vi "ByViServerInterfaceTemplate_4x4x4_CreateClass.vi"(1 "ProjectTreePosition(String or Project Item Ref)":variant, 2 "CreateClassData":T1, 3 "ClassTemplateFolder":path, 5 "error in (no error)":errorcluster, 6 "KeepLvClassRefOpen(False)":bool, 7 "HeaderToApply (take from VIRef or /use 2D-8bit header, Ignored if not wired)":variant) -> (15 "LVClassLibraryRefnum":refnum<vi>, 16 "TemplateVersionUsed":string, 19 "error out":errorcluster)   [LabVIEW 2012]
uses:
  <resource>/Framework/Providers/Open_GDS/ClassProviders/Provider_BaseClassInterface/CreateClassData.ctl
  <resource>/Framework/Providers/Open_GDS/ClassProviders/Common/LvClass_class/GDSLvCLass_ClassSettingsType.ctl
  <resource>/Framework/Providers/Open_GDS/ClassProviders/Common/LvClass_class/GDSLvClass_PlugIn.ctl
  <resource>/Framework/Providers/Open_GDS/ClassProviders/Common/LvClass_class/GDSLvClass_PlugInTypes.ctl
  <resource>/Framework/Providers/Open_GDS/ClassProviders/Provider_BaseClassInterface/ClassWriter_class/ClassWriter.lvclass
  <resource>/Framework/Providers/Open_GDS/ClassProviders/Provider_EndevoGOOP400/ClassWriterGOOP400_class/ClassWriterGOOP400.lvclass
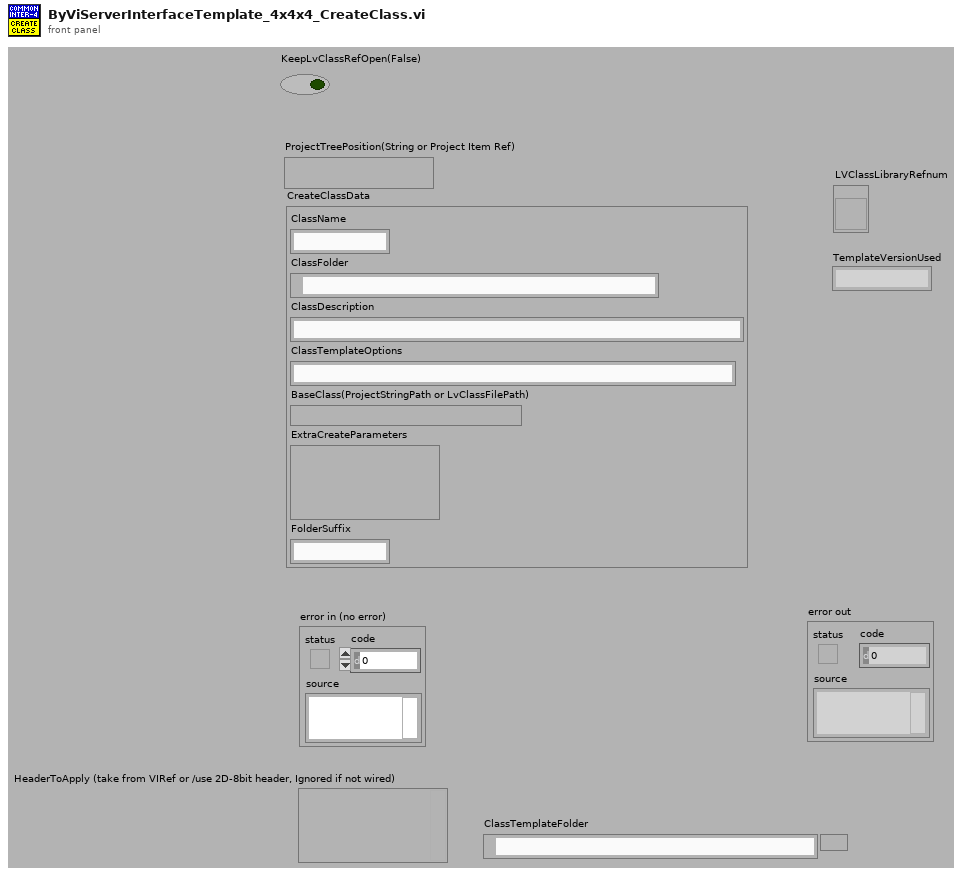
[diagram p1: front panel]
types:
  T1 = typedef "ClassWriter.lvclass/CreateClassData.ctl" = cluster{"ClassName":string, "ClassFolder":path, "ClassDescription":string, "ClassTemplateOptions":string, "BaseClass(ProjectStringPath or LvClassFilePath)":variant, "ExtraCreateParameters":variant, "FolderSuffix":string}
  T2 = cluster{"SubClass":bool, "ClassTemplateFiles":path[], "ClassName":string, "ClassFolder":path, "VIs":refnum<vi>[], "TemplateFolder":path, "ViSubDirs":string[], "TemplateName":string, "BaseClassFolder":path, "RootBaseClassFolder":path, "LvClassPath":path, "ClassRefnum":refnum<vi>, "ProjectRefnum":refnum<vi>, "LvClassFolderPath":path, "BaseClassName":string, "ClassItems":refnum<vi>[], "ViLocked":bool[], "ProjectItemOwner":refnum<vi>, "DeleteFiles":path[], "VIsBefore":refnum<vi>[], "BaseClassPath":path, "BaseConstructorBase":path, "TemplBaseConstructorBase":path, "TemplatePath":path, "TemplateVersion":string, "TemplateParentClass":refnum<vi>, "App":refnum<vi>, "Parent Class":refnum<vi>, "ParentVIs":refnum<vi>[], "TempClass":refnum<vi>}
  T3 = typedef "GDSLvCLass_ClassSettingsType.ctl" = cluster{"ClassProviderName":string, "ClassTemplateUsed":string, "ClassTemplateVersion":string, "ClassDescription":string, "PlugIns":T4[], "ConnectorPanePattern":string}
  T4 = typedef "GDSLvClass_PlugIn.ctl" = cluster{"Type":T5, "ID":string, "Version":string, "Path":path, "Name":string, "Data":variant}
  T5 = typedef "GDSLvClass_PlugInTypes.ctl" = enum16{"DesignPattern", "MethodTypes"}
  T6 = enum32{"invalid lock state", "Not Locked", "Locked (No Password)", "Password-protected"}
  T7 = cluster{"Major":u16, "Minor":u16, "Fix":u16, "Build":u16}
  T8 = typedef "Scripting_ConnectorPanePatternType.ctl" = u16
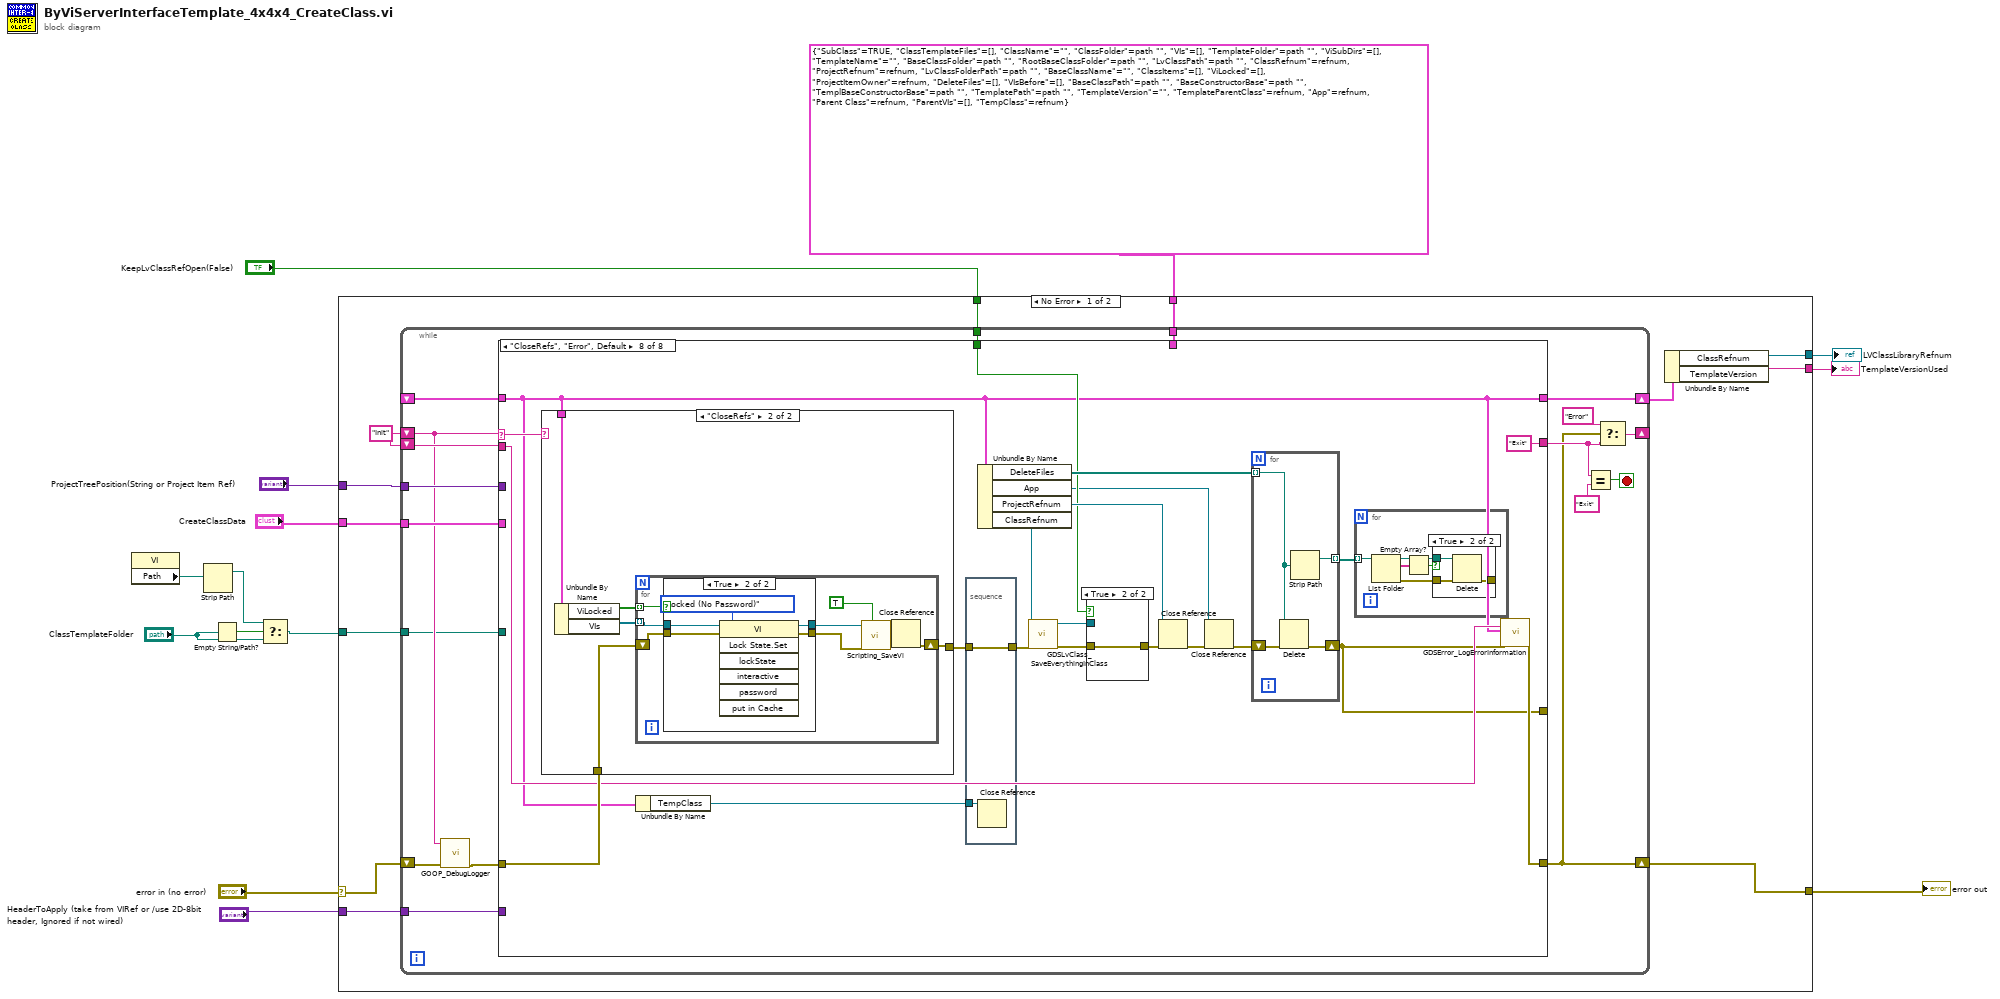
[diagram p0: block diagram]
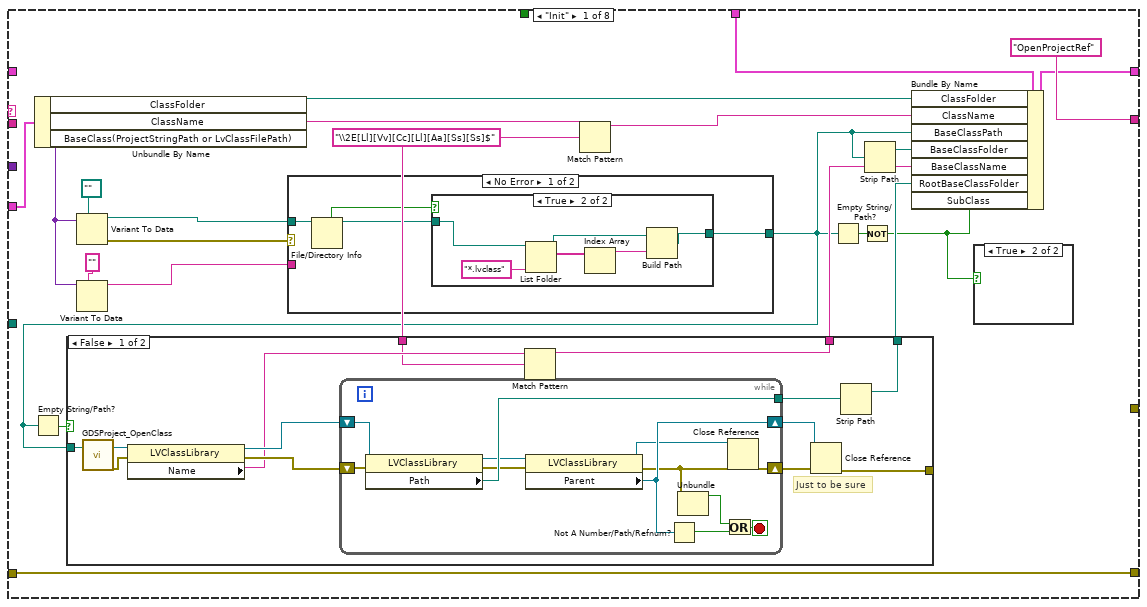
[diagram p2: hidden frame]
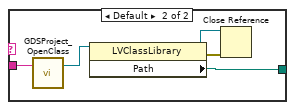
[diagram p7: hidden frame]
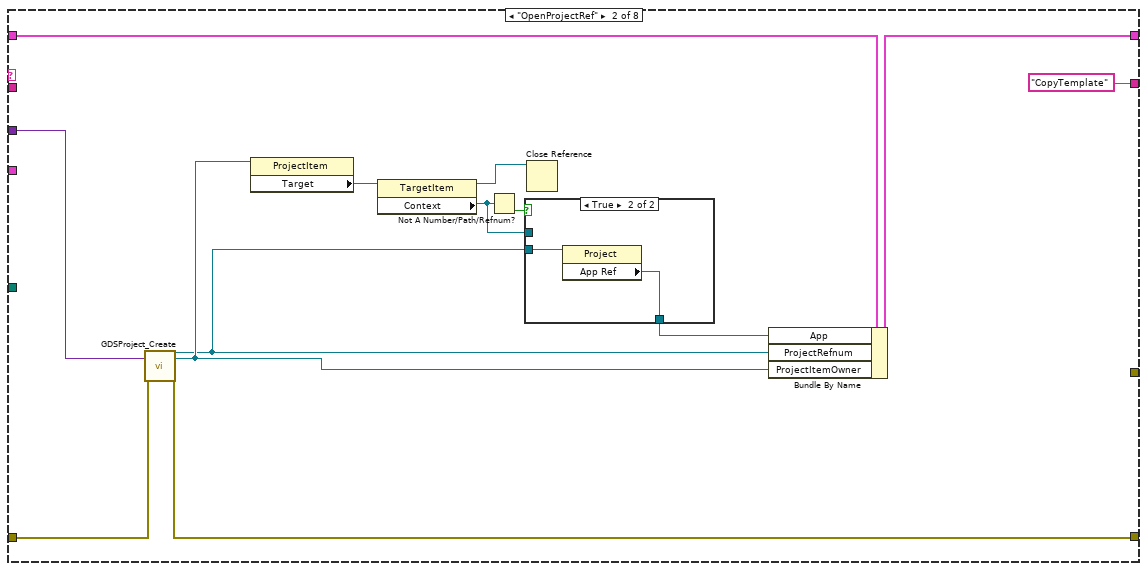
[diagram p8: hidden frame]
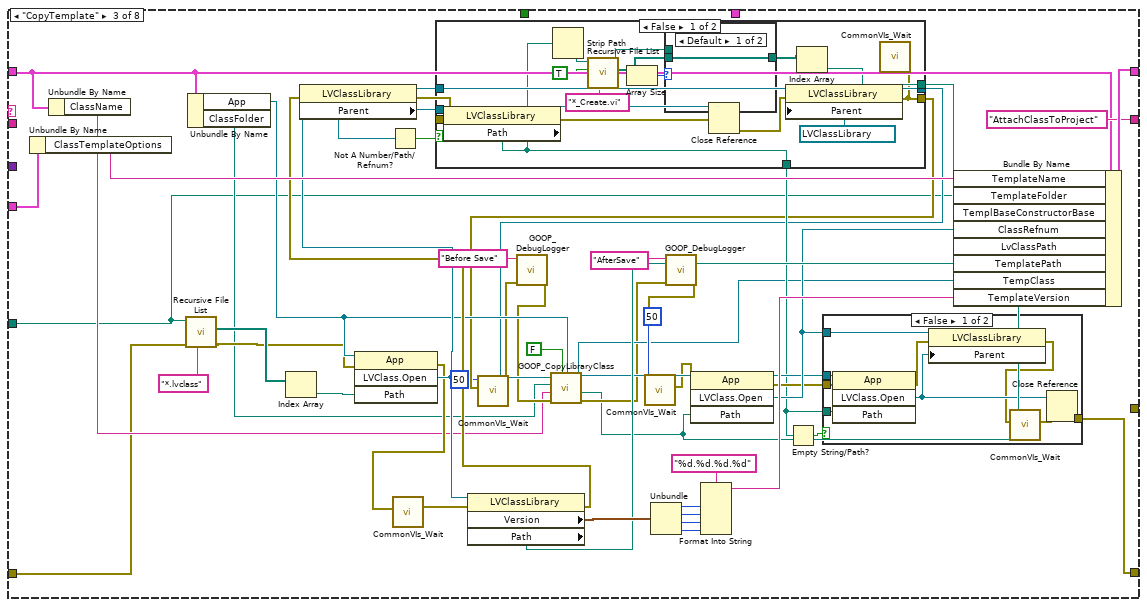
[diagram p10: hidden frame]
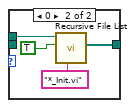
[diagram p12: hidden frame]
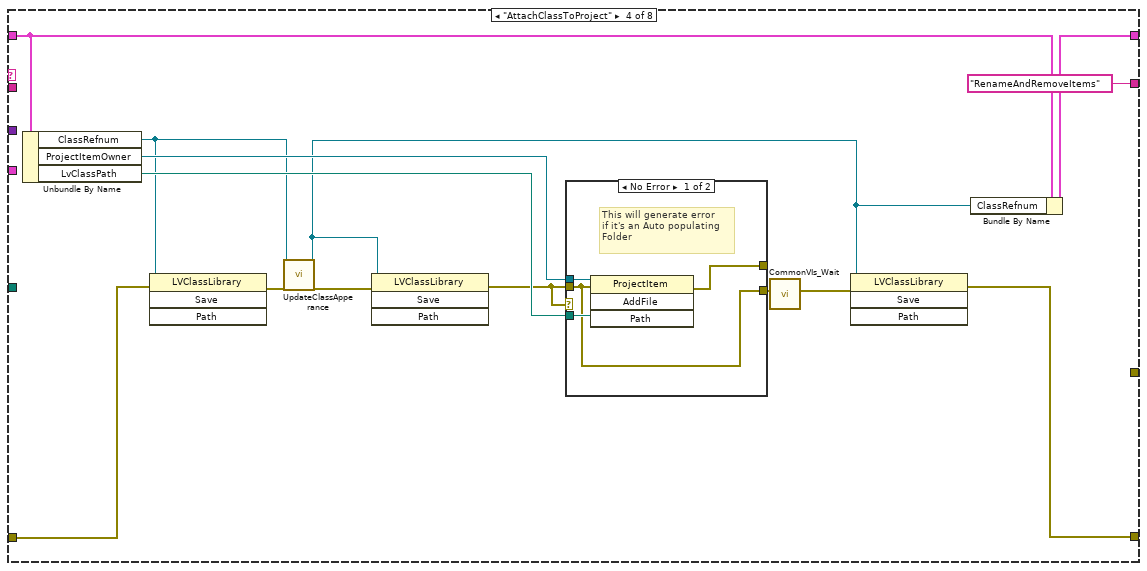
[diagram p14: hidden frame]
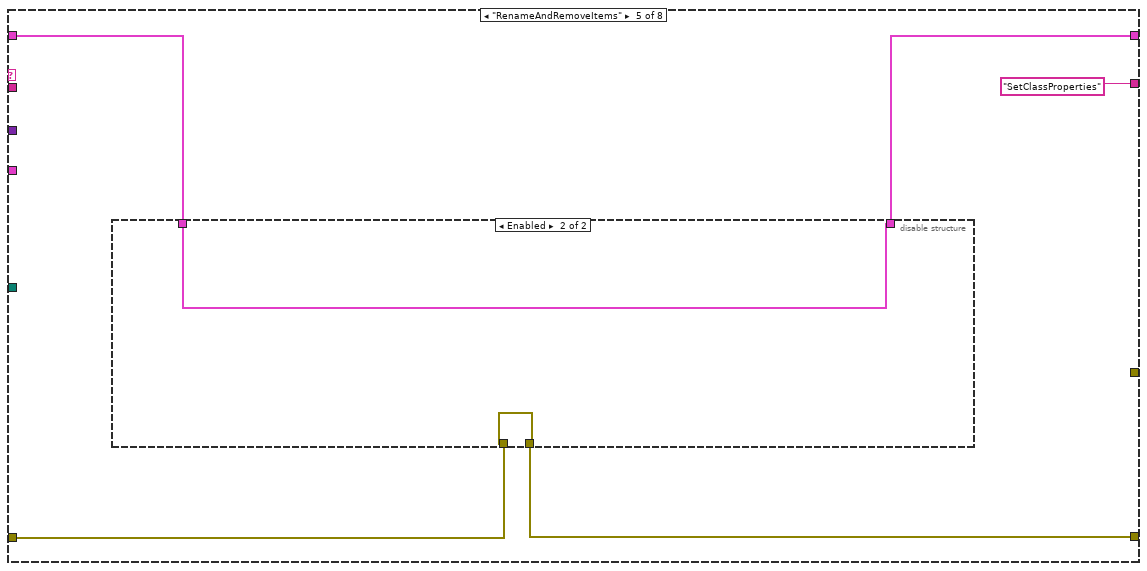
[diagram p16: hidden frame]
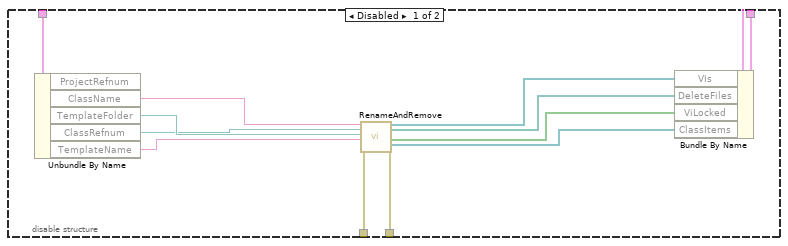
[diagram p17: hidden frame]
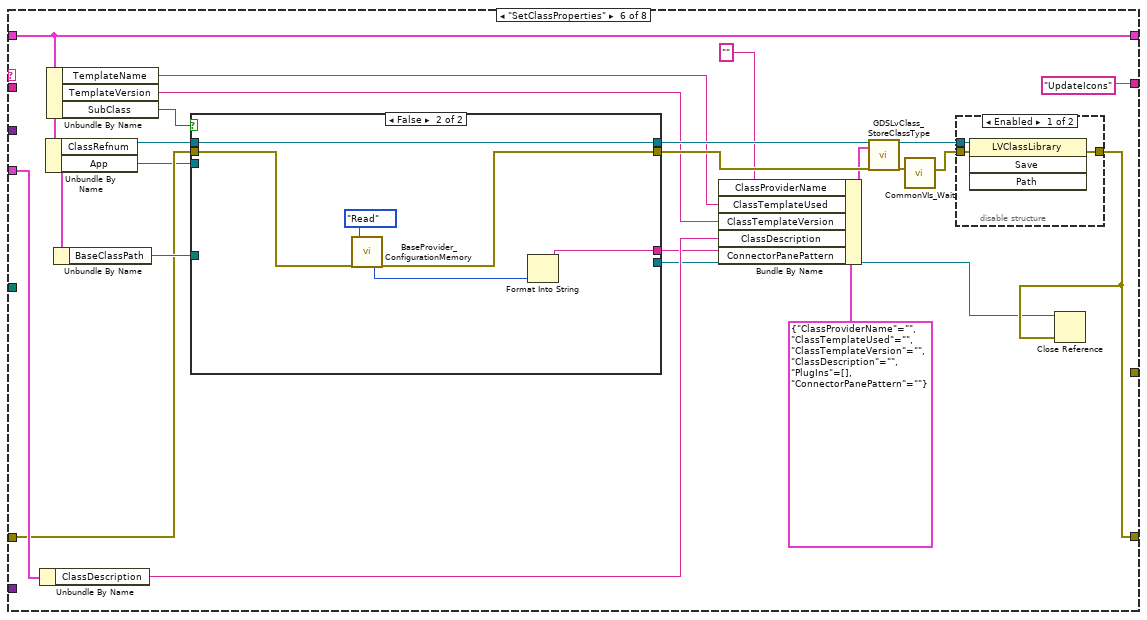
[diagram p18: hidden frame]
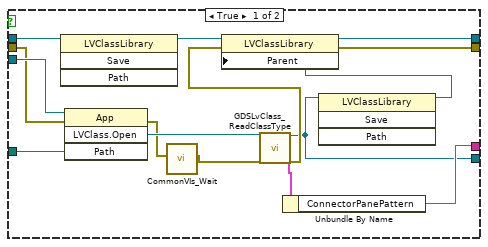
[diagram p20: hidden frame]
diagram:
  n1 = property class="VI"() -> ("Path"=w5:path)  [unwired: 2 in, 2 out]
  n2 = Strip Path(path=w5) -> (stripped path=w2:path)  [unwired: 1 out]
  n3 = Empty String/Path?(string/path="ClassTemplateFolder") -> (empty?=w4:bool)
  n4 = Select(t=w2, s=w4, f="ClassTemplateFolder") -> (s? t:f=w1:path)
  n5 = case shown="No Error" "error in (no error)" {
    selector: "error in (no error)" -> [w17 w368]
    tunnel: [w26 w368] -> w12
    tunnel: "ProjectTreePosition(String or Project Item Ref)" -> [w25 _]
    tunnel: "CreateClassData" -> [w24 _]
    tunnel: "HeaderToApply (take from VIRef or /use 2D-8bit header, Ignored if not wired)" -> [w23 _]
    tunnel: "KeepLvClassRefOpen(False)" -> [w22 _]
    tunnel: [w21 _] -> w7
    tunnel: [w20 _] -> w6
    tunnel: T2 {"SubClass"=TRUE, "ClassTemplateFiles"=[], "ClassName"="", "ClassFolder"=path "", "VIs"=[], "TemplateFolder"=path "", "ViSubDirs"=[], "TemplateName"="", "BaseClassFolder"=path "", "RootBaseClassFolder"=path "", "LvClassPath"=path "", "ClassRefnum"=refnum, "ProjectRefnum"=refnum, "LvClassFolderPath"=path "", "BaseClassName"="", "ClassItems"=[], "ViLocked"=[], "ProjectItemOwner"=refnum, "DeleteFiles"=[], "VIsBefore"=[], "BaseClassPath"=path "", "BaseConstructorBase"=path "", "TemplBaseConstructorBase"=path "", "TemplatePath"=path "", "TemplateVersion"="", "TemplateParentClass"=refnum, "App"=refnum, "Parent Class"=refnum, "ParentVIs"=[], "TempClass"=refnum} ("output cluster") -> [w19 _]
    tunnel: w1 -> [w15 _]
    frame No Error {
      w16 = "Init" ("t")
      n6 = while {
        shift-right: [w36] -> w26
        shift-left: w17 -> [w30]
        shift-right: [w40] -> _
        shift-left: w16 -> [w28]
        shift-right: [w43] -> w18
        shift-left: _ -> [w44]
        tunnel: w19 -> [w38]
        tunnel: w25 -> [w35]
        tunnel: w24 -> [w34]
        shift-left: w16 -> [w33]
        tunnel: w23 -> [w32]
        tunnel: w22 -> [w31]
        tunnel: w15 -> [w27]
        stop <- w41 stop-if-true
        n7 = call <resource>:"GOOP_DebugLogger.vi"("error in (no error)"=w30, "State"=w28) -> ("error out"=w29:errorcluster)  [unwired: 9 in]
        n8 = case shown="\"CloseRefs\", \"Error\", Default" w28 {
          selector: w28 -> [_ _ _ _ _ _ _ w323]
          tunnel: w44 -> [_ w120 w170 w223 w233 w259 w303 w307]
          tunnel: [w63 w119 w175 w222 w234 w259 w303 w307] -> w43
          tunnel: w29 -> [w66 w118 w125 w217 w231 w260 w297 w324]
          tunnel: [w66 w116 w145 w213 w232 w251 w298 w320] -> w36
          tunnel: ["OpenProjectRef" "CopyTemplate" "AttachClassToProject" "RenameAndRemoveItems" "SetClassProperties" "UpdateIcons" "CloseRefs" "Exit"] -> w37
          tunnel: w38 -> [w59 _ _ _ _ _ _ _]
          tunnel: w35 -> [_ w117 _ _ _ _ _ _]
          tunnel: w34 -> [w58 _ w169 _ _ w266 _ _]
          tunnel: w33 -> [_ _ _ _ _ _ _ w319]
          tunnel: w32 -> [_ _ _ _ _ _ w301 _]
          tunnel: w31 -> [_ _ _ _ _ _ _ w315]
          tunnel: [_ _ _ _ _ _ _ w313] -> _
          tunnel: w27 -> [_ _ w126 _ _ _ _ _]
          frame "Init" {
            w55 = "\\2E[Ll][Vv][Cc][Ll][Aa][Ss][Ss]$" ("regular expression")
            n9 = Unbundle By Name(w58) -> ("ClassFolder"=w52:path, "ClassName"=w51:string, "BaseClass(ProjectStringPath or LvClassFilePath)"=w57:variant)
            n10 = Variant To Data(type=path "" ("path"), Variant=w57) -> (data=w48:path, error out=w49:errorcluster)  [unwired: 1 in]
            n11 = Variant To Data(type="" ("regular expression"), Variant=w57) -> (data=w60:string)  [unwired: 1 in, 1 out]
            n12 = case shown="No Error" w49 {
              tunnel: [w94 w102] -> w46
              tunnel: w60 -> [_ w103]
              tunnel: w48 -> [w93 _]
              frame No Error {
                n13 = File/Directory Info(path=w93) -> (path out=w91:path, directory=w92:bool)  [unwired: 1 in, 5 out]
                n14 = case shown="True" w92 {
                  tunnel: [w95 w97] -> w94
                  tunnel: w91 -> [w95 w96]
                  frame False {
                  }
                  frame True {
                    n15 = List Folder(path=w96, pattern="*.lvclass") -> (path out=w98:path, filenames=w100:string[])  [unwired: 2 in, 2 out]
                    n16 = Index Array(array=w100) -> (element=w99:string)  [unwired: 1 in]
                    n17 = Build Path(base path=w98, name or relative path=w99) -> (appended path=w97:path)
                  }
                }
              }
              frame Error {
                n18 = case shown="\"\"" w103 {
                  tunnel: w103 -> [_ w108]
                  tunnel: [_ w104] -> w102
                  frame "" {
                  }
                  frame Default {
                    n19 = call <resource>:"GDSProject_OpenClass.vi"("ClassPath(FilePath/ProjectTreePath/LvCLassRef)"=w108) -> ("LVClass.Open"=w107:refnum<vi>)  [unwired: 16 in, 2 out]
                    n20 = property class="LVClassLibrary"(reference=w107) -> (reference out=w105:refnum<vi>, error out=w106:errorcluster, "Path"=w104:path)  [unwired: 1 in]
                    n21 = Close Reference(reference=w105, error in (no error)=w106) -> ()  [unwired: 1 out]
                  }
                }
              }
            }
            n22 = Empty String/Path?(string/path=w46) -> (empty?=w53:bool)
            n23 = case shown="False" w53 {
              tunnel: [w76 _] -> w56
              tunnel: w55 -> [w70 _]
              tunnel: [w69 _] -> w54
              tunnel: w46 -> [w68 _]
              tunnel: [w67 _] -> _
              frame False {
                # "Just to be sure"
                n24 = call <resource>:"GDSProject_OpenClass.vi"("ClassPath(FilePath/ProjectTreePath/LvCLassRef)"=w68) -> ("LVClass.Open"=w73:refnum<vi>, "error out"=w75:errorcluster)  [unwired: 16 in, 1 out]
                n25 = property class="LVClassLibrary"(reference=w73, error in=w75) -> (reference out=w72:refnum<vi>, error out=w74:errorcluster, "Name"=w71:string)
                n26 = while {
                  shift-right: [w87] -> w79
                  shift-left: w74 -> [w82]
                  shift-right: [w88] -> w78
                  shift-left: w72 -> [w90]
                  tunnel: [w89] -> w77
                  stop <- w84 stop-if-true
                  n27 = property class="LVClassLibrary"(reference=w90, error in=w82) -> (reference out=w80:refnum<vi>, error out=w81:errorcluster, "Path"=w89:path)
                  n28 = property class="LVClassLibrary"(reference=w80, error in=w81) -> (reference out=w83:refnum<vi>, error out=w87:errorcluster, "Parent"=w88:refnum<vi>)
                  n29 = Not A Number/Path/Refnum?(number/path/refnum=w88) -> (NaN/Path/Refnum?=w85:bool)
                  n30 = Unbundle(w87) -> ("status"=w86:bool)  [unwired: 2 out]
                  n31 = Or(x=w86, y=w85) -> (x .or. y?=w84:bool)
                  n32 = Close Reference(reference=w83) -> ()  [unwired: 1 in, 1 out]
                }
                n33 = Match Pattern(string=w71, regular expression=w70) -> (before substring=w69:string)  [unwired: 1 in, 3 out]
                n34 = Close Reference(reference=w78, error in (no error)=w79) -> (error out=w67:errorcluster)
                n35 = Strip Path(path=w77) -> (stripped path=w76:path)  [unwired: 1 out]
              }
              frame True {
              }
            }
            n36 = Match Pattern(string=w51, regular expression=w55) -> (before substring=w64:string)  [unwired: 1 in, 3 out]
            n37 = Empty String/Path?(string/path=w46) -> (empty?=w47:bool)
            n38 = Not(x=w47) -> (.not. x?=w45:bool)
            n39 = Strip Path(path=w46) -> (stripped path=w50:path)  [unwired: 1 out]
            n40 = Bundle By Name(cluster=w59, "ClassFolder"=w52, "ClassName"=w64, "BaseClassPath"=w46, "BaseClassFolder"=w50, "BaseClassName"=w54, "RootBaseClassFolder"=w56, "SubClass"=w45) -> (w63:T2)
            n41 = case shown="True" w45 {
              frame False {
              }
              frame True {
              }
            }
          }
          frame "OpenProjectRef" {
            n42 = call <resource>:"GDSProject_Create.vi"("ProjectTreePosition(String or Project Item Ref)"=w117, "error in (no error)"=w118) -> ("Project Refnum"=w110:refnum<vi>, "Project Item"=w111:refnum<vi>, "error out"=w116:errorcluster)  [unwired: 15 in]
            n43 = property class="ProjectItem"(reference=w111) -> ("Target"=w115:refnum<vi>)  [unwired: 1 in, 2 out]
            n44 = property class="TargetItem"(reference=w115) -> (reference out=w114:refnum<vi>, "Context"=w112:refnum<vi>)  [unwired: 1 in, 1 out]
            n45 = Not A Number/Path/Refnum?(number/path/refnum=w112) -> (NaN/Path/Refnum?=w113:bool)
            n46 = case shown="True" w113 {
              tunnel: [w122 w124] -> w109
              tunnel: w110 -> [_ w123]
              tunnel: w112 -> [w122 _]
              frame False {
              }
              frame True {
                n47 = property class="Project"(reference=w123) -> ("App Ref"=w124:refnum<vi>)  [unwired: 1 in, 2 out]
              }
            }
            n48 = Close Reference(reference=w114) -> ()  [unwired: 1 in, 1 out]
            n49 = Bundle By Name(cluster=w120, "App"=w109, "ProjectRefnum"=w110, "ProjectItemOwner"=w111) -> (w119:T2)
          }
          frame "CopyTemplate" {
            n50 = Unbundle By Name(w169) -> ("ClassTemplateOptions"=w168:string)
            n51 = Unbundle By Name(w170) -> ("ClassName"=w129:string)
            n52 = call <vilib>:"Recursive File List.vi"("pattern"="*.lvclass", "error in (no error)"=w125, "Folder Path"=w126) -> ("error out"=w146:errorcluster, "All Files in Dir"=w172:path[])  [unwired: 4 in, 3 out]
            n53 = Unbundle By Name(w170) -> ("App"=w147:refnum<vi>, "ClassFolder"=w128:path)
            n54 = Index Array(array=w172) -> (element=w171:path)  [unwired: 1 in]
            n55 = invoke class="App" method="LVClass.Open"(reference=w147, error in=w146, "Path"=w171) -> (error out=w142:errorcluster, "LVClass.Open"=w154:refnum<vi>)  [unwired: 1 in, 2 out]
            n56 = call <resource>:"CommonVIs_Wait.vi"("error in"=w142) -> ("error out"=w143:errorcluster)  [unwired: 9 in]
            n57 = property class="LVClassLibrary"(reference=w154, error in=w143) -> (error out=w155:errorcluster, "Version"=w167:T7, "Path"=w161:path)  [unwired: 1 out]
            n58 = property class="LVClassLibrary"(reference=w154, error in=w155) -> (reference out=w159:refnum<vi>, error out=w151:errorcluster, "Parent"=w152:refnum<vi>)
            n59 = Not A Number/Path/Refnum?(number/path/refnum=w152) -> (NaN/Path/Refnum?=w150:bool)
            n60 = case shown="False" w150 {
              tunnel: w159 -> [w200 w209]
              tunnel: [w199 w209] -> w133
              tunnel: [w186 w210] -> w141
              tunnel: [w196 _] -> w153
              tunnel: w152 -> [w194 _]
              tunnel: w151 -> [w193 w210]
              tunnel: [w191 _] -> w149
              frame False {
                n61 = property class="LVClassLibrary"(reference=w194, error in=w193) -> (reference out=w202:refnum<vi>, error out=w203:errorcluster, "Path"=w191:path)
                n62 = Strip Path(path=w191) -> (stripped path=w195:path)  [unwired: 1 out]
                n63 = call <vilib>:"Recursive File List.vi"("pattern"="*_Create.vi", "Treat LLBs as Folders?"=TRUE, "Folder Path"=w195) -> ("All Files in Dir"=w187:path[], "dup Folder Path"=w188:path)  [unwired: 4 in, 3 out]
                n64 = Array Size(array=w187) -> (size(s)=w190:i32)
                n65 = case shown="Default" w190 {
                  tunnel: w187 -> [w204 _]
                  tunnel: [w204 w205] -> w189
                  tunnel: w188 -> [_ w206]
                  frame Default {
                  }
                  frame 0 {
                    n66 = call <vilib>:"Recursive File List.vi"("pattern"="*_Init.vi", "Treat LLBs as Folders?"=TRUE, "Folder Path"=w206) -> ("All Files in Dir"=w205:path[])  [unwired: 4 in, 4 out]
                  }
                }
                n67 = Close Reference(reference=w202, error in (no error)=w203) -> (error out=w201:errorcluster)
                n68 = property class="LVClassLibrary"(reference=w200, error in=w201, "Parent"=refnum<vi> refnum ("Parent Class")) -> (reference out=w199:refnum<vi>, error out=w186:errorcluster)
                n69 = Index Array(array=w189) -> (element=w196:path)  [unwired: 1 in]
                n70 = call <resource>:"CommonVIs_Wait.vi"("error in"=w186) -> ()  [unwired: 9 in, 1 out]
              }
              frame True {
              }
            }
            n71 = call <resource>:"CommonVIs_Wait.vi"("error in"=w141, "Wait(150ms)"=u32 50) -> ("error out"=w138:errorcluster)  [unwired: 8 in]
            n72 = call <resource>:"GOOP_DebugLogger.vi"("error in (no error)"=w138, "State"="Before Save") -> ("error out"=w132:errorcluster)  [unwired: 9 in]
            n73 = call <resource>:"GOOP_CopyLibraryClass.vi"("ManualCopy"=FALSE, "error in"=w132, "New Name"=w129, "Path"=w128, "LVClassIn"=w133) -> ("error out"=w131:errorcluster, "New Lib Path"=w130:path, "LVClassOut"=w134:refnum<vi>)  [unwired: 4 in]
            n74 = Unbundle(w167) -> ("Major"=w165:u16, "Minor"=w164:u16, "Fix"=w163:u16, "Build"=w162:u16)
            n75 = call <resource>:"GOOP_DebugLogger.vi"("error in (no error)"=w131, "State"="AfterSave") -> ("error out"=w136:errorcluster)  [unwired: 9 in]
            n76 = call <resource>:"CommonVIs_Wait.vi"("error in"=w136, "Wait(150ms)"=u32 50) -> ("error out"=w144:errorcluster)  [unwired: 8 in]
            n77 = invoke class="App" method="LVClass.Open"(reference=w147, error in=w144, "Path"=w130) -> (reference out=w157:refnum<vi>, error out=w156:errorcluster, "LVClass.Open"=w158:refnum<vi>)  [unwired: 1 in, 1 out]
            n78 = Format Into String(format string="%d.%d.%d.%d", w165, w164, w163, w162) -> (resulting string=w160:string)  [unwired: 2 in, 1 out]
            n79 = Empty String/Path?(string/path=w149) -> (empty?=w148:bool)
            n80 = case shown="False" w148 {
              tunnel: w158 -> [w184 _]
              tunnel: w157 -> [w183 _]
              tunnel: w156 -> [w182 w185]
              tunnel: [w181 w185] -> w145
              tunnel: w149 -> [w179 _]
              frame False {
                n81 = invoke class="App" method="LVClass.Open"(reference=w183, error in=w182, "Path"=w179) -> (error out=w178:errorcluster, "LVClass.Open"=w180:refnum<vi>)  [unwired: 1 in, 2 out]
                n82 = property class="LVClassLibrary"(reference=w184, error in=w178, "Parent"=w180) -> (error out=w176:errorcluster)  [unwired: 1 out]
                n83 = call <resource>:"CommonVIs_Wait.vi"("error in"=w176) -> ("error out"=w177:errorcluster)  [unwired: 9 in]
                n84 = Close Reference(reference=w180, error in (no error)=w177) -> (error out=w181:errorcluster)
              }
              frame True {
              }
            }
            n85 = Bundle By Name(cluster=w170, "TemplateName"=w168, "TemplateFolder"=w126, "TemplBaseConstructorBase"=w153, "ClassRefnum"=w158, "LvClassPath"=w130, "TemplatePath"=w161, "TempClass"=w134, "TemplateVersion"=w160) -> (w175:T2)
          }
          frame "AttachClassToProject" {
            n86 = Unbundle By Name(w223) -> ("ClassRefnum"=w216:refnum<vi>, "ProjectItemOwner"=w224:refnum<vi>, "LvClassPath"=w220:path)
            n87 = invoke class="LVClassLibrary" method="Save"(reference=w216, error in=w217) -> (error out=w218:errorcluster)  [unwired: 2 in, 3 out]
            n88 = call <resource>:"UpdateClassApperance.vi"("ClassRefIn"=w216, "error in (no error)"=w218) -> ("ClassRefOut"=w211:refnum<vi>, "error out"=w215:errorcluster)  [unwired: 16 in]
            n89 = invoke class="LVClassLibrary" method="Save"(reference=w211, error in=w215) -> (error out=w212:errorcluster)  [unwired: 2 in, 3 out]
            n90 = case shown="No Error" w212 {
              tunnel: w224 -> [w228 _]
              tunnel: w220 -> [w227 _]
              tunnel: [w226 w229] -> w219
              tunnel: w212 -> [w226 w229]
              tunnel: [w225 _] -> _
              frame No Error {
                # "This will generate error\nif it's an Auto populating\nFolder"
                n91 = invoke class="ProjectItem" method="AddFile"(reference=w228, error in=w226, "Path"=w227) -> (error out=w225:errorcluster)  [unwired: 1 in, 3 out]
              }
              frame Error {
              }
            }
            n92 = call <resource>:"CommonVIs_Wait.vi"("error in"=w219) -> ("error out"=w214:errorcluster)  [unwired: 9 in]
            n93 = invoke class="LVClassLibrary" method="Save"(reference=w211, error in=w214) -> (error out=w213:errorcluster)  [unwired: 2 in, 3 out]
            n94 = Bundle By Name(cluster=w223, "ClassRefnum"=w211) -> (w222:T2)
          }
          frame "RenameAndRemoveItems" {
            n95 = disable-structure shown="Enabled" {
              disable-tunnel: [w244 w247] -> w234
              disable-tunnel: w233 -> [w242 w247]
              disable-tunnel: [w240 w248] -> w232
              disable-tunnel: w231 -> [w239 w248]
              frame Disabled {
                n96 = Unbundle By Name(w242) -> ("ClassName"=w246:string, "TemplateFolder"=w243:path, "ClassRefnum"=w241:refnum<vi>, "TemplateName"=w235:string)  [unwired: 1 out]
                n97 = call <resource>:"RenameAndRemove.vi"("ClassName"=w246, "ClassRefnum"=w241, "TemplateFolder"=w243, "TemplateName"=w235, "error in"=w239) -> ("ViRefsOut"=w245:refnum<vi>[], "DeleteFiles"=w238:path[], "ItemLocked"=w237:bool[], "Items"=w236:refnum<vi>[], "error out"=w240:errorcluster)  [unwired: 10 in]
                n98 = Bundle By Name(cluster=w242, "VIs"=w245, "DeleteFiles"=w238, "ViLocked"=w237, "ClassItems"=w236) -> (w244:T2)
              }
              frame Enabled {
              }
            }
          }
          frame "SetClassProperties" {
            n99 = Unbundle By Name(w266) -> ("ClassDescription"=w263:string)
            n100 = Unbundle By Name(w259) -> ("ClassRefnum"=w261:refnum<vi>, "App"=w256:refnum<vi>)
            n101 = Unbundle By Name(w259) -> ("TemplateName"=w262:string, "TemplateVersion"=w257:string, "SubClass"=w270:bool)
            n102 = Unbundle By Name(w259) -> ("BaseClassPath"=w269:path)
            n103 = case shown="False" w270 {
              tunnel: w261 -> [w278 w295]
              tunnel: [w289 w295] -> w268
              tunnel: w260 -> [w282 w291]
              tunnel: [w288 w290] -> w267
              tunnel: w269 -> [w287 _]
              tunnel: w256 -> [w283 _]
              tunnel: [w284 w292] -> w255
              tunnel: [w276 _] -> w250
              frame True {
                n104 = invoke class="LVClassLibrary" method="Save"(reference=w278) -> (reference out=w277:refnum<vi>)  [unwired: 3 in, 3 out]
                n105 = invoke class="App" method="LVClass.Open"(reference=w283, error in=w282, "Path"=w287) -> (error out=w281:errorcluster, "LVClass.Open"=w286:refnum<vi>)  [unwired: 1 in, 2 out]
                n106 = call <resource>:"CommonVIs_Wait.vi"("error in"=w281) -> ("error out"=w280:errorcluster)  [unwired: 9 in]
                n107 = call <resource>:"GDSLvClass_ReadClassType.vi"("Class Refnum In"=w286, "error in (no error)"=w280) -> ("Class Refnum Out"=w276:refnum<vi>, "ClassSettings"=w285:T3, "error out"=w279:errorcluster)  [unwired: 15 in]
                n108 = Unbundle By Name(w285) -> ("ConnectorPanePattern"=w284:string)
                n109 = invoke class="LVClassLibrary" method="Save"(reference=w276) -> (reference out=w275:refnum<vi>)  [unwired: 3 in, 3 out]
                n110 = property class="LVClassLibrary"(reference=w277, error in=w279, "Parent"=w275) -> (reference out=w289:refnum<vi>, error out=w288:errorcluster)
              }
              frame False {
                n111 = call <resource>:"BaseProvider_ConfigurationMemory.vi"("error in (no error)"=w291, "Action"=enum16{"Read", "Load", "Save"}."Read") -> ("PatternOut"=w294:T8, "error out"=w290:errorcluster)  [unwired: 11 in, 5 out]
                n112 = Format Into String(w294) -> (resulting string=w292:string)  [unwired: 3 in, 1 out]
              }
            }
            n113 = Bundle By Name(cluster=T3 {"ClassProviderName"="", "ClassTemplateUsed"="", "ClassTemplateVersion"="", "ClassDescription"="", "PlugIns"=[], "ConnectorPanePattern"=""} ("ClassSettings"), "ClassProviderName"="", "ClassTemplateUsed"=w262, "ClassTemplateVersion"=w257, "ClassDescription"=w263, "ConnectorPanePattern"=w255) -> (w264:T3)
            n114 = call <resource>:"GDSLvClass_StoreClassType.vi"("Class Refnum In"=w268, "ClassSettings"=w264, "error in (no error)"=w267) -> ("Class Refnum Out"=w254:refnum<vi>, "error out"=w253:errorcluster)  [unwired: 15 in]
            n115 = call <resource>:"CommonVIs_Wait.vi"("error in"=w253) -> ("error out"=w252:errorcluster)  [unwired: 9 in]
            n116 = disable-structure shown="Enabled" {
              disable-tunnel: [w273 w274] -> w251
              disable-tunnel: w254 -> [w272 _]
              disable-tunnel: w252 -> [w271 w274]
              frame Enabled {
                n117 = invoke class="LVClassLibrary" method="Save"(reference=w272, error in=w271) -> (error out=w273:errorcluster)  [unwired: 2 in, 3 out]
              }
              frame Disabled {
              }
            }
            n118 = Close Reference(reference=w250, error in (no error)=w251) -> ()  [unwired: 1 out]
          }
          frame "UpdateIcons" {
            n119 = Unbundle By Name(w303) -> ("ClassRefnum"=w302:refnum<vi>)
            n120 = Unbundle By Name(w303) -> ("ClassName"=w304:string)  [unwired: 1 out]
            n121 = Empty String/Path?(string/path=w301) -> (empty?=w300:bool)
            n122 = Not(x=w300) -> (.not. x?=w299:bool)
            n123 = call <resource>:"GDSLvIcon_DialogUpdateClass.vi"("ClassPath(FilePath/ProjectTreePath/LvCLassRef)"=w302, "ClassName"=w304, "AutoUpdate"=w299, "error in (no error)"=w297, "HeaderToApply (take from VIRef or /use 2D-8bit header, Ignored if not wired)"=w301) -> ("error out"=w298:errorcluster)  [unwired: 14 in]
          }
          frame "CloseRefs", "Error", Default {
            n124 = case shown="\"CloseRefs\"" w323 {
              tunnel: w324 -> [w346 w350]
              tunnel: w307 -> [w345 w349]
              tunnel: [w346 w348] -> w308
              frame "False", Default {
                n125 = Unbundle By Name(w345) -> ("VIs"=w344:refnum<vi>[])
                n126 = Close Reference(reference=w344) -> ()  [unwired: 1 in, 1 out]
              }
              frame "CloseRefs" {
                n127 = Unbundle By Name(w349) -> ("ViLocked"=w347:bool[], "VIs"=w351:refnum<vi>[])
                n128 = for {
                  tunnel: w351 -> [w356] mode=indexing
                  shift-right: [w352] -> w348
                  shift-left: w350 -> [w357]
                  tunnel: w347 -> [w353] mode=indexing
                  n129 = case shown="True" w353 {
                    tunnel: w357 -> [w361 w367]
                    tunnel: w356 -> [w362 w366]
                    tunnel: [w361 w365] -> w355
                    tunnel: [w362 w364] -> w354
                    frame False {
                    }
                    frame True {
                      n130 = invoke class="VI" method="Lock State.Set"(reference=w366, error in=w367, "lockState"=T6."Locked (No Password)" ("Lock State")) -> (reference out=w364:refnum<vi>, error out=w365:errorcluster)  [unwired: 4 in, 5 out]
                    }
                  }
                  n131 = call <resource>:"Scripting_SaveVi.vi"("ForceResaving(False)"=TRUE, "error in (no error)"=w355, "VIRefToSaveIn"=w354) -> ("error out"=w360:errorcluster, "VIRefToSaveOut"=w359:refnum<vi>)  [unwired: 7 in]
                  n132 = Close Reference(reference=w359, error in (no error)=w360) -> (error out=w352:errorcluster)
                }
              }
            }
            n133 = Unbundle By Name(w307) -> ("TempClass"=w306:refnum<vi>)
            n134 = stacked-sequence {
              tunnel: w308 -> [w326]
              tunnel: [w326] -> w305
              tunnel: w306 -> [w327]
              frame #0 {
                n135 = Close Reference(reference=w327) -> ()  [unwired: 1 in, 1 out]
              }
            }
            n136 = Unbundle By Name(w307) -> ("DeleteFiles"=w318:path[], "App"=w310:refnum<vi>, "ProjectRefnum"=w321:refnum<vi>, "ClassRefnum"=w317:refnum<vi>)
            n137 = call <resource>:"GDSLvClass_SaveEverythingInClass.vi"("ClassRefIn"=w317, "error in"=w305) -> ("ClassRefOut"=w312:refnum<vi>, "error out"=w314:errorcluster)  [unwired: 16 in]
            n138 = case shown="True" w315 {
              tunnel: [w330 w331] -> w322
              tunnel: w314 -> [w329 w331]
              tunnel: w312 -> [w328 _]
              frame False {
                n139 = Close Reference(reference=w328, error in (no error)=w329) -> (error out=w330:errorcluster)
              }
              frame True {
              }
            }
            n140 = Close Reference(reference=w321, error in (no error)=w322) -> (error out=w311:errorcluster)
            n141 = Close Reference(reference=w310, error in (no error)=w311) -> (error out=w309:errorcluster)
            n142 = for {
              shift-right: [w342] -> w313
              shift-left: w309 -> [w343]
              tunnel: w318 -> [w341] mode=indexing
              tunnel: [w340] -> w316 mode=indexing
              n143 = Delete(path (use dialog)=w341, error in=w343) -> (error out=w342:errorcluster)  [unwired: 3 in, 2 out]
              n144 = Strip Path(path=w341) -> (stripped path=w340:path)  [unwired: 1 out]
            }
            n145 = for {
              tunnel: w316 -> [w336] mode=indexing
              n146 = List Folder(path=w336) -> (path out=w332:path, filenames=w335:string[], error out=w333:errorcluster)  [unwired: 3 in, 1 out]
              n147 = Empty Array?(array=w335) -> (empty?=w334:bool)
              n148 = case shown="True" w334 {
                tunnel: w333 -> [_ w339]
                tunnel: w332 -> [_ w338]
                tunnel: [_ w337] -> _
                frame False {
                }
                frame True {
                  n149 = Delete(path (use dialog)=w338, error in=w339) -> (error out=w337:errorcluster)  [unwired: 3 in, 2 out]
                }
              }
            }
            n150 = call <resource>:"GDSError_LogErrorInformation.vi"("State"=w319, "LocalVariableData"=w307, "error in (no error)"=w313) -> ("error out"=w320:errorcluster)  [unwired: 16 in]
          }
        }
        n151 = Equal?(x=w37, y="Exit") -> (x = y?=w41:bool)
        n152 = Select(t="Error", s=w36, f=w37) -> (s? t:f=w40:string)
      }
      n153 = Unbundle By Name(w18) -> ("ClassRefnum"=w21:refnum<vi>, "TemplateVersion"=w20:string)
    }
    frame Error {
    }
  }
  "error out" <- w12
  "LVClassLibraryRefnum" <- w7
  "TemplateVersionUsed" <- w6
